vi "Mutate_Template.vi"(11 "Input":T1) -> (0 "error out":errorcluster, 3 "Output":T1)   [LabVIEW 2020, in "BlueSerializableTemplate.lvlib" / "BlueSerializableTemplate.lvclass"]
uses:
  BlueSerializableTemplate.lvclass
  SerializableData.ctl
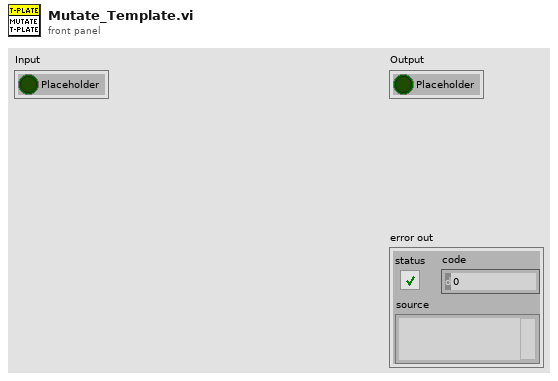
[diagram p1: front panel]
types:
  T1 = typedef "BlueSerializableTemplate.lvlib/BlueSerializableTemplate.lvclass/SerializableData.ctl" = cluster{"Placeholder":bool}
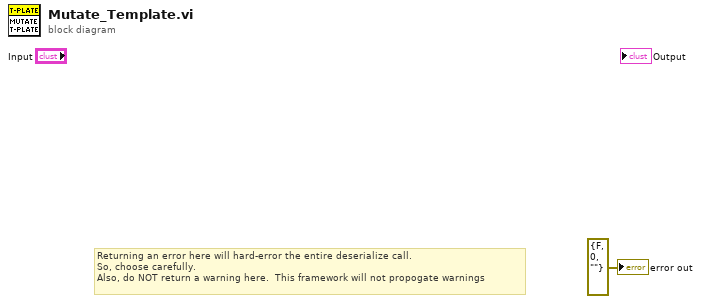
[diagram p0: block diagram]
diagram:
  # "Returning an error here will hard-error the entire deserialize call.\nSo, choose carefully.\nAlso, do NOT return a warning here.  This framework will not propogate warnings"
  "error out" <- errorcluster {"status"=FALSE, "code"=0, "source"=""} ("error out")
